vi "Callback Event(FGV).vi"(6 "Method":enum16{"Destroy", "Put", "Get"}(ring), 8 "error in":errorcluster, 11 "Callback Event Reference In":T1) -> (0 "error out":errorcluster, 3 "Callback Event Reference Out":T1)   [LabVIEW 2018]
uses:
  Function/Data Def/Callback Event Reference.ctl
  System.Speech
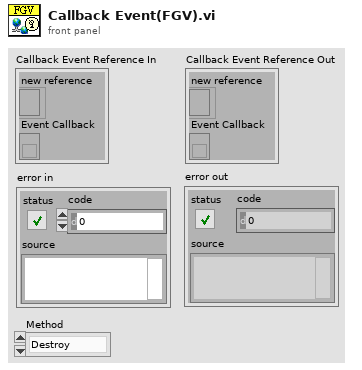
[diagram p1: front panel]
types:
  T1 = typedef "Callback Event Reference.ctl" = cluster{"new reference":refnum<k24>, "Event Callback":refnum<k27>}
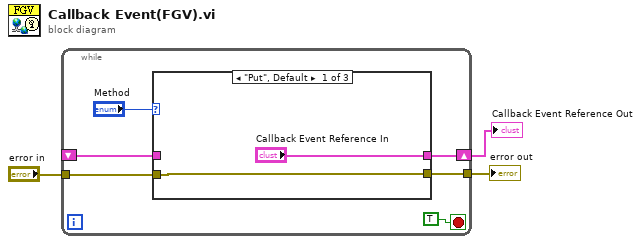
[diagram p0: block diagram]
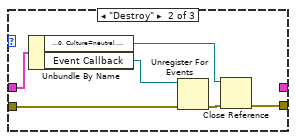
[diagram p2: hidden frame]
diagram:
  n1 = while {
    shift-right: [w7] -> w3
    shift-left: _ -> [w6]
    tunnel: "error in" -> [w5]
    tunnel: [w4] -> w1
    stop <- TRUE stop-if-true
    n2 = case shown="\"Put\", Default" "Method" {
      tunnel: ["Callback Event Reference In" _ w19] -> w7
      tunnel: w6 -> [_ w17 w19]
      tunnel: w5 -> [w10 w13 w18]
      tunnel: [w10 w12 w18] -> w4
      frame "Put", Default {
      }
      frame "Destroy" {
        n3 = Unbundle By Name(w17) -> ("new reference"=w14:refnum<k24>, "Event Callback"=w15:refnum<k27>)
        n4 = Unregister For Events(event registration refnum=w15, error in=w13) -> (error out=w16:errorcluster)
        n5 = Close Reference(reference=w14, error in (no error)=w16) -> (error out=w12:errorcluster)
      }
      frame "Get" {
      }
    }
  }
  "error out" <- w1
  "Callback Event Reference Out" <- w3
